vi "get all by type.vi"(8 "error in (no error)":errorcluster, 10 "Type":refnum<class "system object.lvclass">, 11 "SysObj in":refnum<class "Folder.lvclass">) -> (0 "error out":errorcluster, 2 "All objects":refnum<class "system object.lvclass">[](array[class]), 3 "SysObj out":refnum<class "Folder.lvclass">)   [LabVIEW 2020, in "Folder.lvclass"]
uses:
  Folder.lvclass
  system object/system object.lvclass
  Folder.lvclass/Folder.ctl
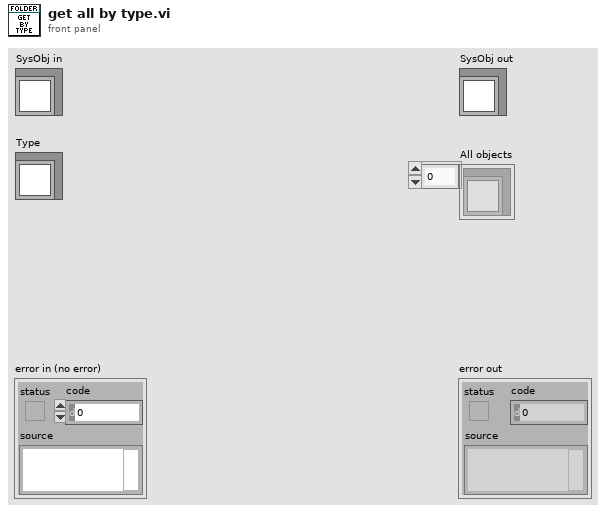
[diagram p1: front panel]
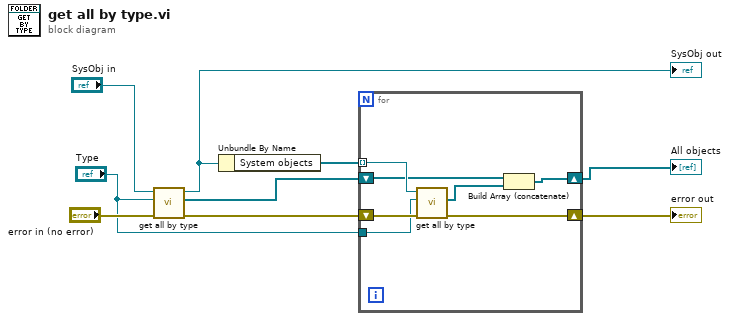
[diagram p0: block diagram]
diagram:
  n1 = call-parent "get all by type.vi"("error in (no error)"="error in (no error)", "Type"="Type", "SysObj in"="SysObj in") -> ("error out"=w4:errorcluster, "All objects"=w5:refnum<class "system object.lvclass">[], "SysObj out"=w7:refnum<class "Folder.lvclass">)  [unwired: 6 in]
  "SysObj out" <- w7
  n2 = Unbundle By Name(w7) -> ("System objects"=w6:refnum<class "system object.lvclass">[])
  n3 = for {
    tunnel: w6 -> [w16] mode=indexing
    shift-right: [w12] -> w1
    shift-left: w5 -> [w14]
    tunnel: "Type" -> [w11]
    shift-right: [w10] -> w2
    shift-left: w4 -> [w15]
    n4 = call-dynamic "get all by type.vi"("error in (no error)"=w15, "Type"=w11, "SysObj in"=w16) -> ("error out"=w10:errorcluster, "All objects"=w13:refnum<class "system object.lvclass">[])  [unwired: 6 in, 1 out]
    n5 = Build Array (concatenate)(w14, w13) -> (w12:refnum<class "system object.lvclass">[])
  }
  "error out" <- w2
  "All objects" <- w1
